vi "send.vi"() -> ()   [LabVIEW 2015]
uses:
  <vilib>/Instr/_visa.llb/VISA Configure Serial Port (Instr).vi
panel:
  out "进度":dbl format="%.2f"
  in  "发送":bool
  in  "文件路径":path
  in  "VISA资源名称":refnum<visa-resource-name>
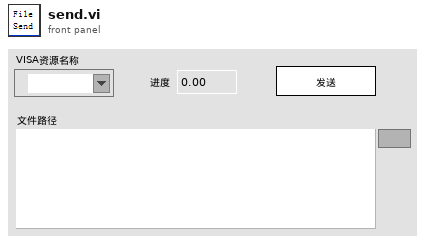
[diagram p1: front panel]
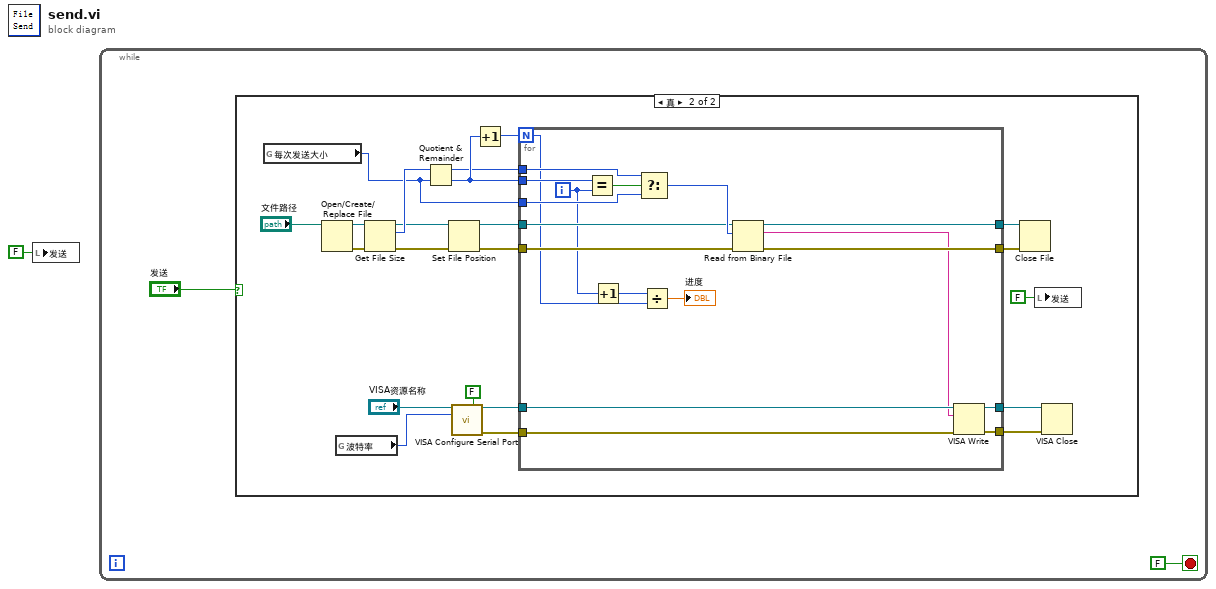
[diagram p0: block diagram]
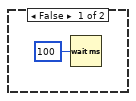
[diagram p2: hidden frame]
diagram:
  n1 = local write "发送"(FALSE ("发送")) -> ()
  n2 = while {
    stop <- FALSE stop-if-true
    n3 = case shown="真" "发送" {
      frame False {
        n4 = Wait (ms)(milliseconds to wait=u32 100 ("等待时间（毫秒）")) -> ()  [unwired: 1 out]
      }
      frame True {
        n5 = global read "全局变量.vi" "每次发送大小"() -> (w5:i32)
        n6 = Open/Create/Replace File(file path (use dialog)="文件路径") -> (refnum out=w17:refnum<file>, error out=w18:errorcluster)  [unwired: 5 in, 1 out]
        n7 = global read "全局变量.vi" "波特率"() -> (w6:u32)
        n8 = Get File Size(file=w17, error in=w18) -> (refnum out=w11:refnum<file>, size (in bytes)=w16:i64, 0:w9:errorcluster)
        n9 = Quotient & Remainder(x=w16, y=w5) -> (x-y*floor(x/y)=w13:i64, floor(x/y)=w15:i64)
        n10 = Set File Position(refnum=w11, error in=w9) -> (refnum out=w10:refnum<file>, error out=w8:errorcluster)  [unwired: 2 in]
        n11 = call-poly "VISA Configure Serial Port"("VISA resource name"="VISA资源名称", "Enable Termination\nChar (T)"=FALSE ("Enable Termination\nChar (T)"), "baud rate (9600)"=w6) -> ("VISA resource name out"=w25:refnum<visa-resource-name>, "error out"=w24:errorcluster)  [unwired: 11 in]
        n12 = Increment(x=w15) -> (x+1=w14:i64)
        n13 = for {
          N: w14 -> [w29]
          tunnel: w25 -> [w40]
          tunnel: w24 -> [w39]
          tunnel: [w44] -> w21
          tunnel: [w43] -> w20
          tunnel: w10 -> [w32]
          tunnel: w8 -> [w31]
          tunnel: [w42] -> w23
          tunnel: [w41] -> w22
          tunnel: w5 -> [w35]
          tunnel: w15 -> [w38]
          tunnel: w13 -> [w36]
          i -> [w30]
          n14 = Equal?(x=w38, y=w30) -> (x = y?=w37:bool)
          n15 = Increment(x=w30) -> (x+1=w27:i32)
          n16 = Select(t=w36, s=w37, f=w35) -> (s? t:f=w34:i64)
          n17 = Divide(x=w27, y=w29) -> (x/y=→"进度":dbl)
          n18 = Read from Binary File(8:w31, 10:w34, 11:w32) -> (0:w41:errorcluster, 2:w33:string, 3:w42:refnum<file>)  [unwired: 3 in, 1 out]
          n19 = VISA Write(VISA resource name=w40, write buffer=w33, error in (no error)=w39) -> (VISA resource name out=w44:refnum<visa-resource-name>, error out=w43:errorcluster)  [unwired: 1 out]
        }
        n20 = Close File(refnum=w23, error in=w22) -> ()  [unwired: 2 out]
        n21 = local write "发送"(FALSE ("发送")) -> ()
        n22 = VISA Close(VISA resource name=w21, error in (no error)=w20) -> ()  [unwired: 1 out]
      }
    }
  }
